vi "Day1_2-3.vi"() -> ()   [LabVIEW 2014]
panel:
  out "배열":dbl[](array[numeric])
  out "숫자(0에서 1)":dbl
  out "웨이브폼 차트":dbl[](graph)
  out "Waveform graph":dbl[](graph)
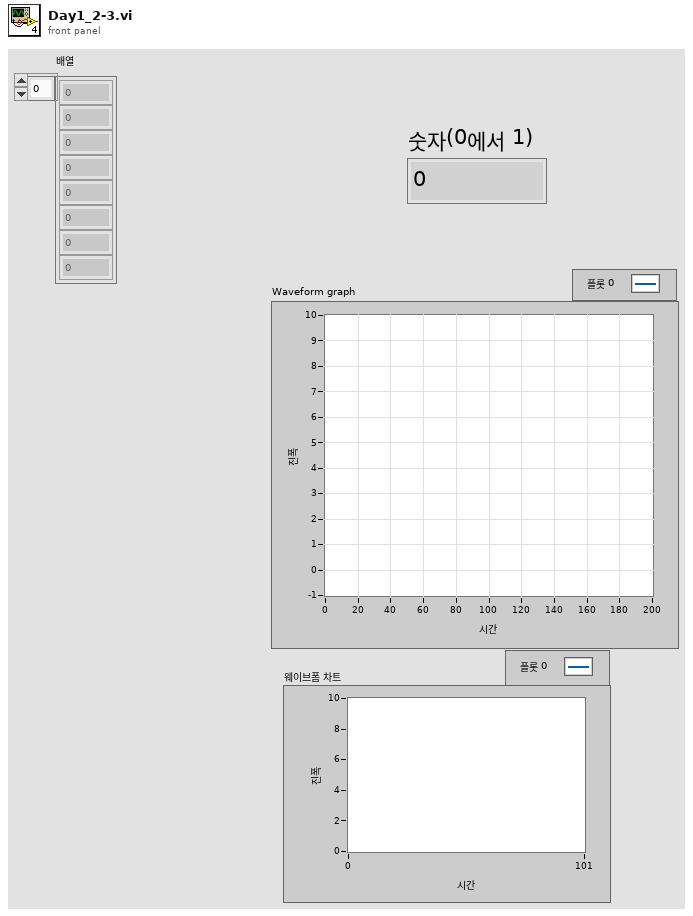
[diagram p1: front panel]
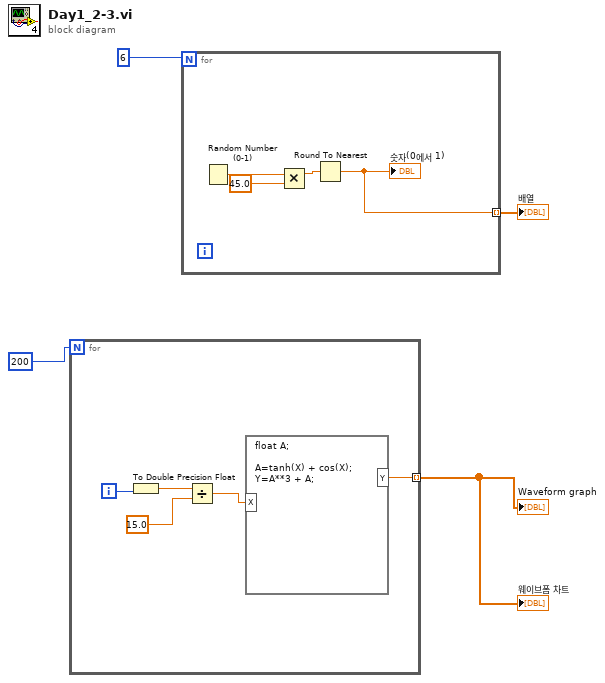
[diagram p0: block diagram]
diagram:
  n1 = for {
    N: 200 -> [_]
    tunnel: [w5] -> w3 mode=indexing
    i -> [w9]
    n2 = To Double Precision Float(number=w9) -> (double precision float=w8:dbl)
    n3 = Divide(x=w8, y=15.0) -> (x/y=w6:dbl)
    n4 = formula code="float A;\n\nA=tanh(X) + cos(X);\nY=A**3 + A;"("X"=w6) -> ("Y"=w5:dbl)
  }
  "Waveform graph" <- w3
  "웨이브폼 차트" <- w3
  n5 = for {
    N: 6 -> [_]
    tunnel: [w10] -> w1 mode=indexing
    n6 = Random Number (0-1)() -> (number: 0 to 1=w13:dbl)
    n7 = Multiply(x=w13, y=45.0) -> (x*y=w12:dbl)
    n8 = Round To Nearest(number=w12) -> (nearest integer value=w10:dbl)
    "숫자(0에서 1)" <- w10
  }
  "배열" <- w1
